vi "Get AI Data Value.vi"(6 "Raw? (false)":bool, 8 "error in (no error)":errorcluster, 10 "AI IOName":string, 11 "DAQ":refnum<class "DAQ.lvclass">) -> (0 "error out":errorcluster, 1 "Timestamp (DBL)":dbl, 2 "Value":dbl, 3 "DAQ":refnum<class "DAQ.lvclass">, 5 "Time Stamp":timestamp)   [LabVIEW 2022 SP3, in "DAQ.lvclass"]
doc: "Developed by Kevin Thompson\nkevin@thompsonengineering.net\n\nCopyright 2018-2020\nThompson Engineering, LLC"
uses:
  DAQ.lvclass
  Process/ProcessSupport/TD DaqThread--enum.ctl
  DAQ.lvclass/DAQ.ctl
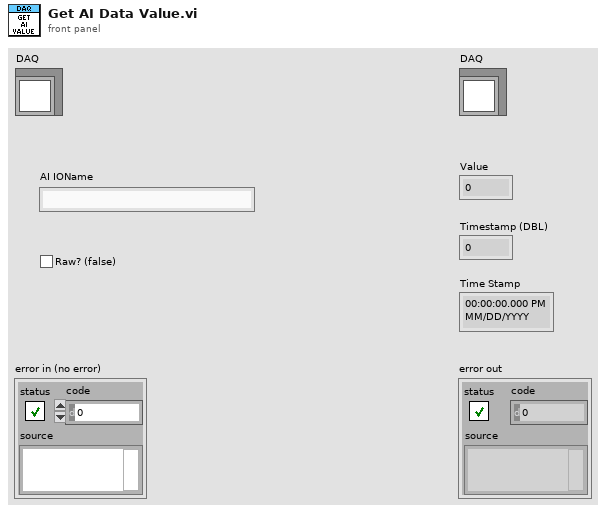
[diagram p1: front panel]
types:
  T1 = typedef "DAQ.lvclass/TD DaqThread--enum.ctl" = enum16{"AI", "DI"}
  T2 = typedef "TD Dynamic CVT DVR--ref.ctl" = refnum<data-value>
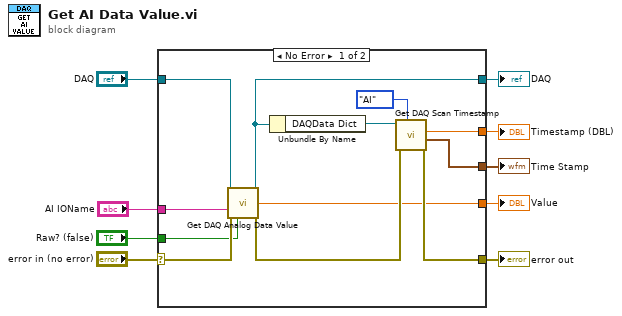
[diagram p0: block diagram]
diagram:
  n1 = case shown="No Error" "error in (no error)" {
    selector: "error in (no error)" -> [w21 w23]
    tunnel: [w16 w23] -> w8
    tunnel: [w19 w22] -> w6
    tunnel: "DAQ" -> [w20 w22]
    tunnel: [w14 _] -> w4
    tunnel: [w13 _] -> w5
    tunnel: [w12 _] -> w3
    tunnel: "Raw? (false)" -> [w11 _]
    tunnel: "AI IOName" -> [w10 _]
    frame No Error {
      n2 = call "Get DAQ Analog Data Value.vi"("DAQ"=w20, "Name"=w10, "error in (no error)"=w21, "Raw? (false)"=w11) -> ("DAQ"=w19:refnum<class "DAQ.lvclass">, "Value"=w12:dbl, "error out"=w17:errorcluster)  [unwired: 9 in]
      n3 = Unbundle By Name(w19) -> ("DAQData Dict"=w18:T2)
      n4 = call "Get DAQ Scan Timestamp.vi"("Daq Thread"=TD_DaqThread--enum."AI", "error in (no error)"=w17, "DaqData dCVT"=w18) -> ("error out"=w16:errorcluster, "Time Stamp"=w13:timestamp, "Timestamp (DBL)"=w14:dbl)  [unwired: 5 in, 1 out]
    }
    frame Error {
    }
  }
  "error out" <- w8
  "DAQ" <- w6
  "Value" <- w3
  "Time Stamp" <- w5
  "Timestamp (DBL)" <- w4
